vi "_Open_Port.vi"(8 "error in (no error)":errorcluster, 11 "Postgres Connector.lvclass":refnum<class "Postgres Connector.lvclass">) -> (0 "error out":errorcluster, 3 "output cluster":refnum<class "Postgres Connector.lvclass">)   [LabVIEW 2019, in "PG_LIB.lvlib" / "Postgres Connector.lvclass"]
doc: "Establish a TCP connection with the server where the database is installed."
uses:
  Postgres Connector.lvclass
  Postgres Connector.lvclass/Postgres Connector.ctl
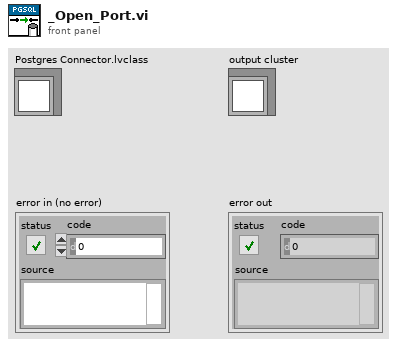
[diagram p1: front panel]
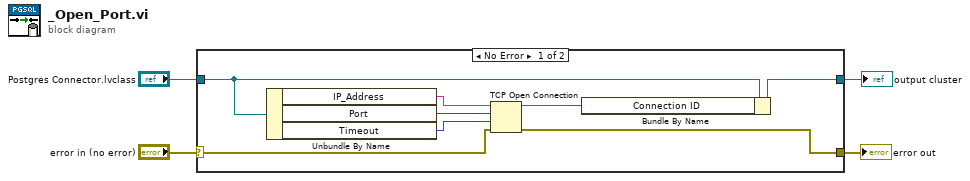
[diagram p0: block diagram]
diagram:
  n1 = case shown="No Error" "error in (no error)" {
    selector: "error in (no error)" -> [w6 w14]
    tunnel: "Postgres Connector.lvclass" -> [w9 w13]
    tunnel: [w7 w13] -> w3
    tunnel: [w5 w14] -> w2
    frame No Error {
      n2 = Unbundle By Name(w9) -> ("IP_Address"=w11:string, "Port"=w12:u16, "Timeout"=w10:i32)
      n3 = TCP Open Connection(address=w11, remote port or service name=w12, timeout ms (60000)=w10, error in (no error)=w6) -> (connection ID=w8:refnum<k5>, error out=w5:errorcluster)  [unwired: 1 in]
      n4 = Bundle By Name(cluster=w9, "Connection ID"=w8) -> (w7:refnum<class "Postgres Connector.lvclass">)
    }
    frame Error {
    }
  }
  "error out" <- w2
  "output cluster" <- w3
